vi "Configure.vi"(8 "error in (no error)":errorcluster, 10 "Iterator Settings":T1={"Prepare timeout (ms)"=200, "Iterate timeout (ms)"=50, "Conclude timeout (ms)"=200, "Iterate period (ms)"=200, "Number of iterations"=5, "Stop Condition"=enum."None", "Time before stop (ms)"=5, "Prepare Msg"=refnum, "Iterate Msg"=refnum, "Conclude Msg"=refnum, "Error Handler"=refnum}, 11 "Iterator Actor in":refnum<class "Iterator Actor.lvclass">) -> (0 "error out":errorcluster, 3 "Iterator Actor out":refnum<class "Iterator Actor.lvclass">)   [LabVIEW 2016, in "Iterator Actor.lvlib" / "Iterator Actor.lvclass"]
doc: "Configures the parameters of the Iterator and starts the sequence."
uses:
  Iterator Actor.lvclass
  Iterator Settings.ctl
  Iterator Actor Messages/Iterator Reply Msg/Iterator Reply Msg.lvclass
  Iterator Actor Messages/Iterator Report Error Msg/Iterator Report Error Msg.lvclass
  Stop Condition.ctl
  Iterator Actor.lvclass/Iterator Actor.ctl
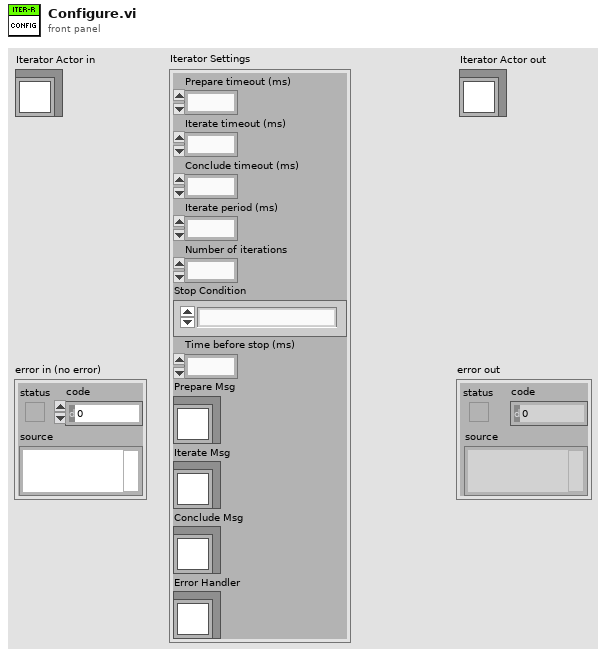
[diagram p1: front panel]
types:
  T1 = typedef "Iterator Actor.lvlib/Iterator Actor.lvclass/Iterator Settings.ctl" = cluster{"Prepare timeout (ms)":i32, "Iterate timeout (ms)":i32, "Conclude timeout (ms)":i32, "Iterate period (ms)":i32, "Number of iterations":i32, "Stop Condition":T2, "Time before stop (ms)":i32, "Prepare Msg":refnum<class "Iterator Reply Msg.lvclass">, "Iterate Msg":refnum<class "Iterator Reply Msg.lvclass">, "Conclude Msg":refnum<class "Iterator Reply Msg.lvclass">, "Error Handler":refnum<class "Iterator Report Error Msg.lvclass">}
  T2 = typedef "Iterator Actor.lvlib/Iterator Actor.lvclass/Stop Condition.ctl" = enum16{"None", "Number of iterations", "Time elapsed", "Iteration result"}
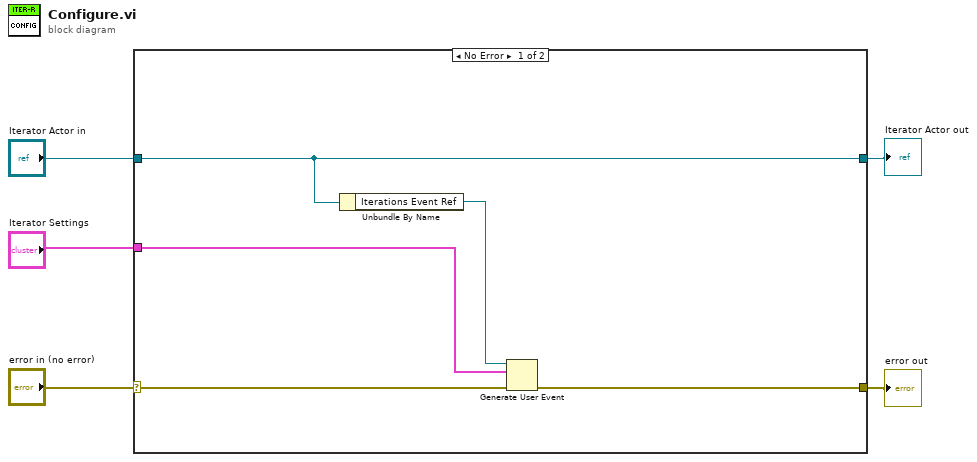
[diagram p0: block diagram]
diagram:
  n1 = case shown="No Error" "error in (no error)" {
    selector: "error in (no error)" -> [w10 w12]
    tunnel: [w9 w12] -> w4
    tunnel: [w8 w11] -> w2
    tunnel: "Iterator Actor in" -> [w8 w11]
    tunnel: "Iterator Settings" -> [w7 _]
    frame No Error {
      n2 = Unbundle By Name(w8) -> ("Iterations Event Ref"=w6:refnum<user-event>)
      n3 = Generate User Event(user event=w6, event data cluster=w7, error in=w10) -> (error out=w9:errorcluster)  [unwired: 1 in, 1 out]
    }
    frame Error {
    }
  }
  "error out" <- w4
  "Iterator Actor out" <- w2
